vi "Stop Manger.vi"(0 "Stop (F)":bool, 1 "Reset":bool) -> (2 "Loop Stop":bool)   [LabVIEW 2012]
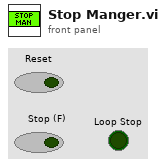
[diagram p1: front panel]
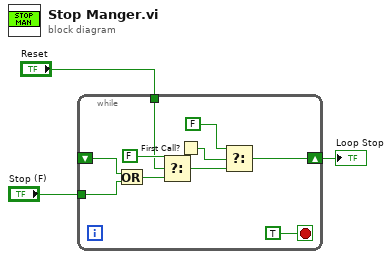
[diagram p0: block diagram]
diagram:
  n1 = while {
    shift-right: [w5] -> w3
    shift-left: _ -> [w10]
    tunnel: "Reset" -> [w11]
    tunnel: "Stop (F)" -> [w9]
    stop <- TRUE stop-if-true
    n2 = Or(x=w10, y=w9) -> (x .or. y?=w8:bool)
    n3 = Select(t=FALSE, s=w11, f=w8) -> (s? t:f=w6:bool)
    n4 = First Call?() -> (First Call?: T/F=w7:bool)
    n5 = Select(t=FALSE, s=w7, f=w6) -> (s? t:f=w5:bool)
  }
  "Loop Stop" <- w3
